vi "set_get_resolution.vi"(8 "error in (no error)":errorcluster, 10 "Input: Resolution - H/L":string="\r", 11 "StageMG100204SutterMP285 in":refnum<class "StageMG100204SutterMP285.lvclass">=refnum) -> (0 "error out":errorcluster, 3 "StageMG100204SutterMP285 out":refnum<class "StageMG100204SutterMP285.lvclass">)   [LabVIEW 2010, in "StageMG100204SutterMP285.lvclass"]
uses:
  StageMG100204SutterMP285.lvclass
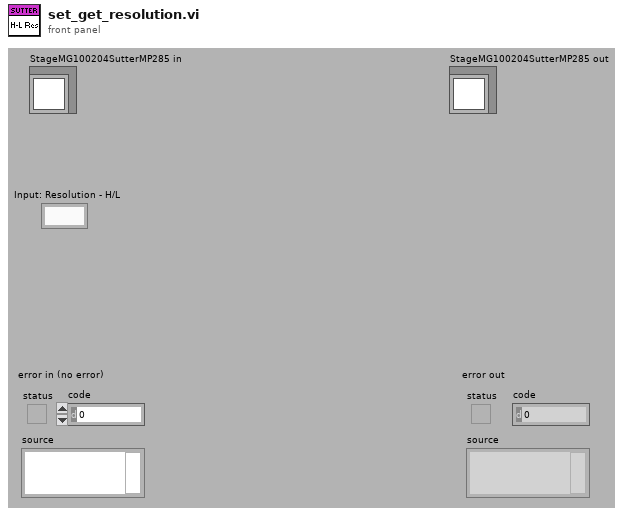
[diagram p1: front panel]
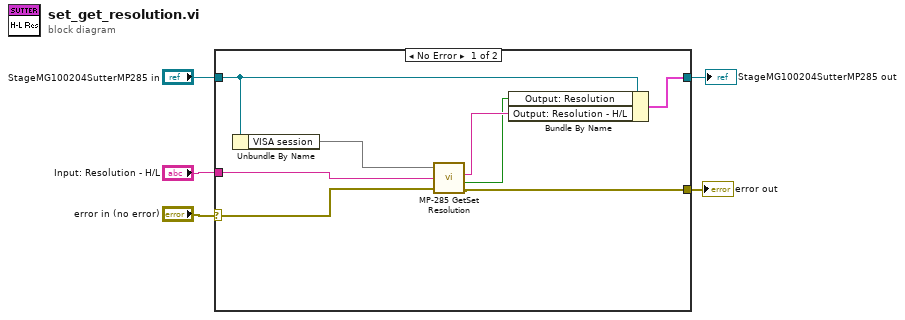
[diagram p0: block diagram]
diagram:
  n1 = case shown="No Error" "error in (no error)" {
    selector: "error in (no error)" -> [w13 w14]
    tunnel: "StageMG100204SutterMP285 in" -> [w9 w15]
    tunnel: [w8 w15] -> w1
    tunnel: [w12 w14] -> w4
    tunnel: "Input: Resolution - H/L" -> [w10 _]
    frame No Error {
      n2 = Unbundle By Name(w9) -> ("VISA session"=w11)
      n3 = call "MP-285 GetSet Resolution.vi"("VISA resource name"=w11, "Input: Resolution - H/L"=w10, "error in (no error)"=w13) -> ("Output: Resolution - H/L"=w7:string, "Output: Resolution"=w6:bool, "error out"=w12:errorcluster)  [unwired: 1 out]
      n4 = Bundle By Name(cluster=w9, "Output: Resolution"=w6, "Output: Resolution - H/L"=w7) -> (w8:cluster{})
    }
    frame Error {
    }
  }
  "error out" <- w4
  "StageMG100204SutterMP285 out" <- w1
